vi "Write SPI Engine.vi"(8 "error in (no error)":errorcluster, 10 "SPI Engine":path, 11 "Bus Configuration in":refnum<class "Bus Configuration.lvclass">) -> (0 "error out":errorcluster, 3 "Bus Configuration out":refnum<class "Bus Configuration.lvclass">)   [LabVIEW 2014, in "Bus Configuration.lvclass"]
uses:
  Bus Configuration.lvclass
  Bus Configuration.lvclass/Bus Configuration.ctl
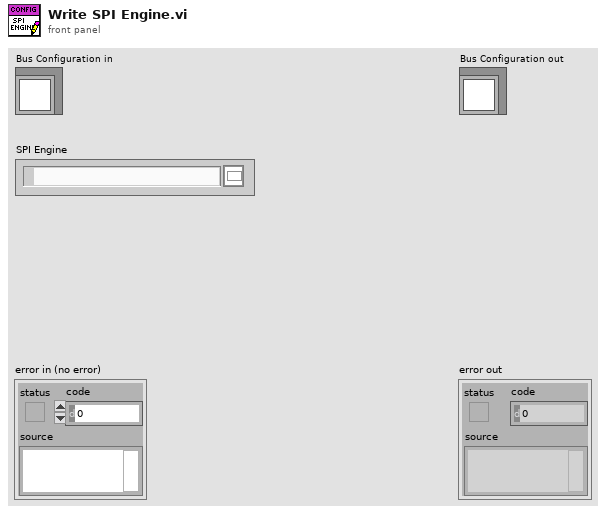
[diagram p1: front panel]
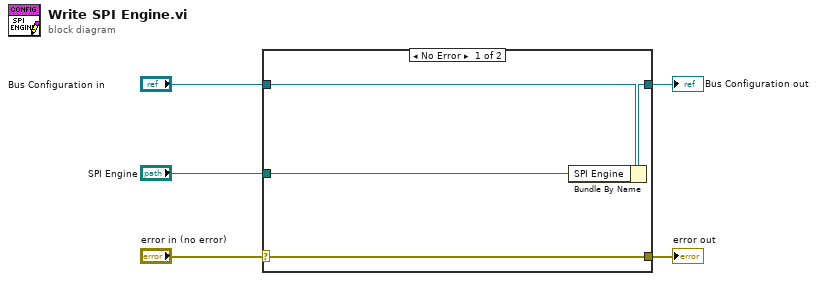
[diagram p0: block diagram]
diagram:
  n1 = case shown="No Error" "error in (no error)" {
    selector: "error in (no error)" -> [w9 w10]
    tunnel: [w9 w10] -> w4
    tunnel: [w7 w11] -> w2
    tunnel: "Bus Configuration in" -> [w8 w11]
    tunnel: "SPI Engine" -> [w6 _]
    frame No Error {
      n2 = Bundle By Name(cluster=w8, "SPI Engine"=w6) -> (w7:refnum<class "Bus Configuration.lvclass">)
    }
    frame Error {
    }
  }
  "error out" <- w4
  "Bus Configuration out" <- w2
